vi "writeDataFile.vi"(8 "error in (no error)":errorcluster, 10 "WriteDataFileInput":T1, 11 "ITestLog in":refnum<class "ITestLog.lvclass">) -> (0 "error out":errorcluster, 2 "Relative Path":string, 3 "ITestLog out":refnum<class "ITestLog.lvclass">)   [LabVIEW 2015, in "ITestLog.lvclass"]
uses:
  ITestLog.lvclass
  Typedefs/WriteDataFileInput.ctl
  Typedefs/FAMTTypedefs.lvlib
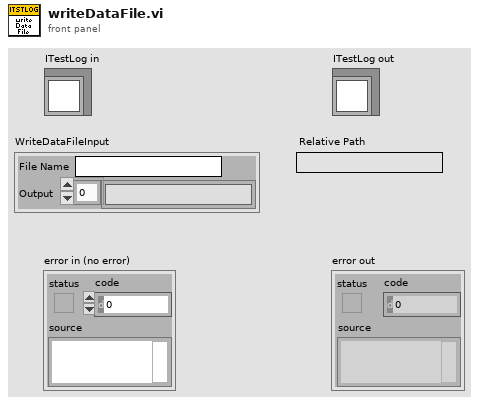
[diagram p1: front panel]
types:
  T1 = typedef "FAMTTypedefs.lvlib/WriteDataFileInput.ctl" = cluster{"File Name":string, "Output":string[]}
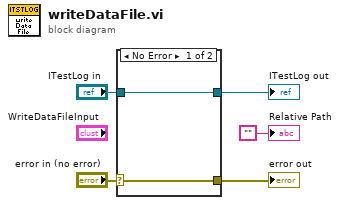
[diagram p0: block diagram]
diagram:
  n1 = case shown="No Error" "error in (no error)" {
    selector: "error in (no error)" -> [w6 w9]
    tunnel: [w6 w9] -> w5
    tunnel: [w7 w8] -> w3
    tunnel: "ITestLog in" -> [w7 w8]
    frame No Error {
    }
    frame Error {
    }
  }
  "error out" <- w5
  "ITestLog out" <- w3
  "Relative Path" <- ""
